vi "Save File General Main File Save Configuration Path.vi"(8 "Error In":errorcluster, 11 "Tool Base Path":path) -> (0 "Error Out":errorcluster, 1 "Appliance Previous Run Path":path, 2 "Calibration File Path":path, 3 "File Save Configuration Data Path":path, 5 "DOE Capacity Path":path)   [LabVIEW 2018, in "File Setup.lvlib"]
uses:
  File Setup.lvlib
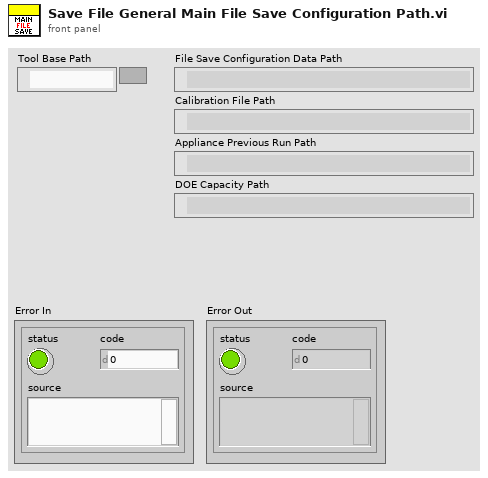
[diagram p1: front panel]
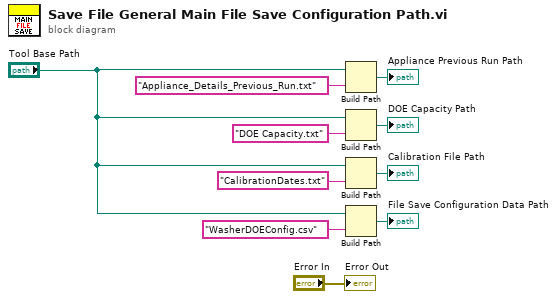
[diagram p0: block diagram]
diagram:
  n1 = Build Path(base path="Tool Base Path", name or relative path="Appliance_Details_Previous_Run.txt") -> (appended path=→"Appliance Previous Run Path":path)
  n2 = Build Path(base path="Tool Base Path", name or relative path="DOE Capacity.txt") -> (appended path=→"DOE Capacity Path":path)
  n3 = Build Path(base path="Tool Base Path", name or relative path="CalibrationDates.txt" ("string")) -> (appended path=→"Calibration File Path":path)
  n4 = Build Path(base path="Tool Base Path", name or relative path="WasherDOEConfig.csv" ("string")) -> (appended path=→"File Save Configuration Data Path":path)
  "Error Out" <- "Error In"
